vi "Motion Path Planing Sub_VI.vi"(2 "Motion Planning Inputs":T2) -> (6 "Motion Profile":T3=enum."Triangular", 7 "Motion Planning Outputs":T1)   [LabVIEW 2017]
uses:
  Motion Type Def.ctl
  <vilib>/imath/engines/lvmath2/RunTimeEngine/ArithmeticOperatorToken/NIMS_ArithmeticOperator_power(S).vi
  <instcachedir>/0/NIMS_ArithmeticOperator_power(S)_86B1D76B77564424912EAFCCCC7488ED.lvgen/NIMS_ArithmeticOperator_power(S)_86B1D76B77564424912EAFCCCC7488ED_010.vi
  <vilib>/imathl/engines/lvmath/Functions/Error Handling/Create Error.vi
  <vilib>/imath/engines/lvmath2/RunTimeEngine/NodeEndStatement/NIMS_NodeEndStatement_Output.vi
  <instcachedir>/0/NIMS_NodeEndStatement_Output_53EC0D466D134D7ABD903AC30B43404B.lvgen/NIMS_NodeEndStatement_Output_53EC0D466D134D7ABD903AC30B43404B_009.vi
  <instcachedir>/0/NIMS_NodeEndStatement_Output_53EC0D466D134D7ABD903AC30B43404B.lvgen/NIMS_NodeEndStatement_Output_53EC0D466D134D7ABD903AC30B43404B_001.vi
  <vilib>/imath/engines/lvmath2/RunTimeEngine/ErrorHandling/NIMS_Finalize Error.vi
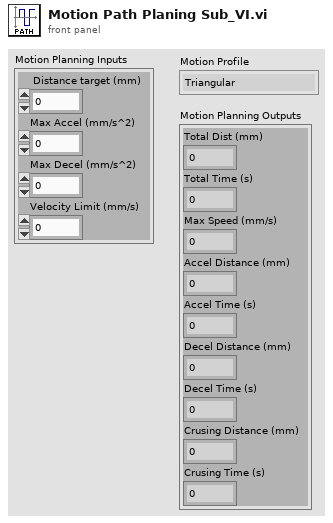
[diagram p1: front panel]
types:
  T1 = cluster{"Crusing Time (s)":dbl, "Decel Time (s)":dbl, "Accel Time (s)":dbl, "Total Time (s)":dbl, "Accel Distance (mm)":dbl, "Decel Distance (mm)":dbl, "Crusing Distance (mm)":dbl, "Total Dist (mm)":dbl, "Max Speed (mm/s)":dbl}
  T2 = cluster{" Distance target (mm)":dbl, "Max Accel (mm/s^2)":dbl, "Max Decel (mm/s^2)":dbl, "Velocity Limit (mm/s) ":dbl}
  T3 = typedef "Motion Type Def.ctl" = enum16{"Trapezodial", "Triangular"}
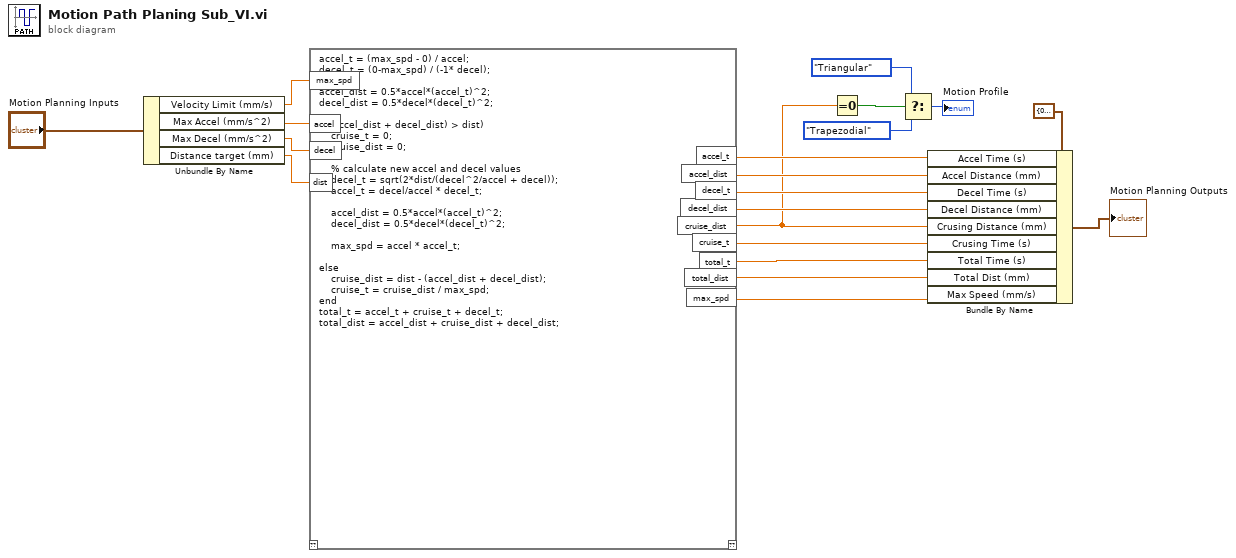
[diagram p0: block diagram]
diagram:
  n1 = Unbundle By Name("Motion Planning Inputs") -> ("Velocity Limit (mm/s)"=w15:dbl, "Max Accel (mm/s^2)"=w13:dbl, "Max Decel (mm/s^2)"=w12:dbl, "Distance target (mm)"=w14:dbl)
  n2 = mathscript code="accel_t = (max_spd - 0) / accel;\ndecel_t = (0-max_spd) / (-1* decel);\n\naccel_dist = 0.5*accel*(accel_t)^2;\ndecel_dist = 0.5*decel*(decel_t)^2;\n\nif((accel_dist + decel_dist) > dist)\n    cruise_t = 0;\n    cruise_dist = 0;\n    \n    % calculate new accel and decel values\n    decel_t = sqrt(2*dist/(decel^2/accel + decel));\n    accel_t = decel/accel * decel_t;\n    \n    accel_dist = 0.5*accel*(accel_t)^2;\n    decel_dist = 0.5*decel*(decel_t)^2;\n    \n    max_spd = accel * accel_t;\n    \nelse\n    cruise_dist = dist - (accel_dist + decel_dist);\n    cruise_t = cruise_dist / max_spd;\nend\ntotal_t = accel_t + cruise_t + decel_t;\ntotal_dist = accel_dist + cruise_dist + decel_dist;"("max_spd"=w15, "dist"=w14, "accel"=w13, "decel"=w12) -> ("accel_dist"=w10:cdb, "accel_t"=w11:cdb, "cruise_dist"=w1:dbl, "cruise_t"=w9:dbl, "decel_dist"=w7:cdb, "decel_t"=w8:cdb, "total_t"=w6:cdb, "total_dist"=w5:cdb, "max_spd"=w2:cdb)  [unwired: 1 in, 1 out]
  n3 = Equal To 0?(x=w1) -> (x = 0?=w16:bool)
  n4 = Select(t=Motion_Type_Def."Triangular", s=w16, f=Motion_Type_Def."Trapezodial") -> (s? t:f=→"Motion Profile":T3)
  n5 = Bundle By Name(cluster=T1 {"Crusing Time (s)"=0.0, "Decel Time (s)"=0.0, "Accel Time (s)"=0.0, "Total Time (s)"=0.0, "Accel Distance (mm)"=0.0, "Decel Distance (mm)"=0.0, "Crusing Distance (mm)"=0.0, "Total Dist (mm)"=0.0, "Max Speed (mm/s)"=0.0} ("Motion Planning Outputs"), "Accel Time (s)"=w11, "Accel Distance (mm)"=w10, "Decel Time (s)"=w8, "Decel Distance (mm)"=w7, "Crusing Distance (mm)"=w1, "Crusing Time (s)"=w9, "Total Time (s)"=w6, "Total Dist (mm)"=w5, "Max Speed (mm/s)"=w2) -> (→"Motion Planning Outputs":T1)
